vi "Configure.vi"(8 "error in (no error)":errorcluster, 10 "ConfigRef In":T1, 11 "Temperature Device in":refnum<class "Temperature Device.lvclass">) -> (0 "error out":errorcluster, 3 "Temperature Device out":refnum<class "Temperature Device.lvclass">)   [LabVIEW 2015, in "Temperature Device.lvclass"]
uses:
  Temperature Device.lvclass
  <vilib>/Utility/config.llb/Config Data RefNum.ctl
  <vilib>/Utility/config.llb/NI_LVConfig.lvlib
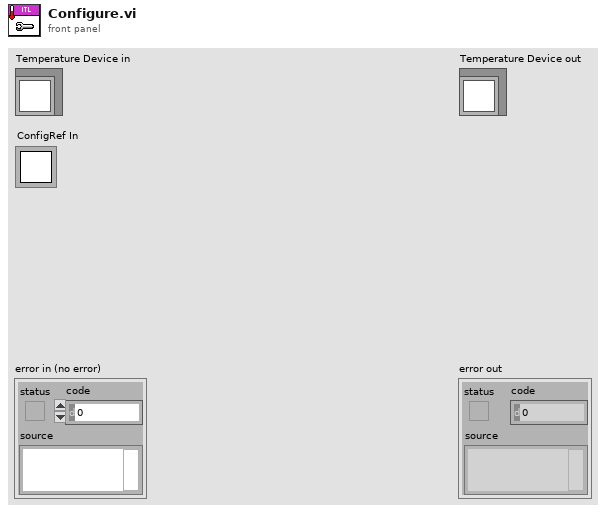
[diagram p1: front panel]
types:
  T1 = typedef "NI_LVConfig.lvlib/Config Data RefNum.ctl" = refnum<k1>
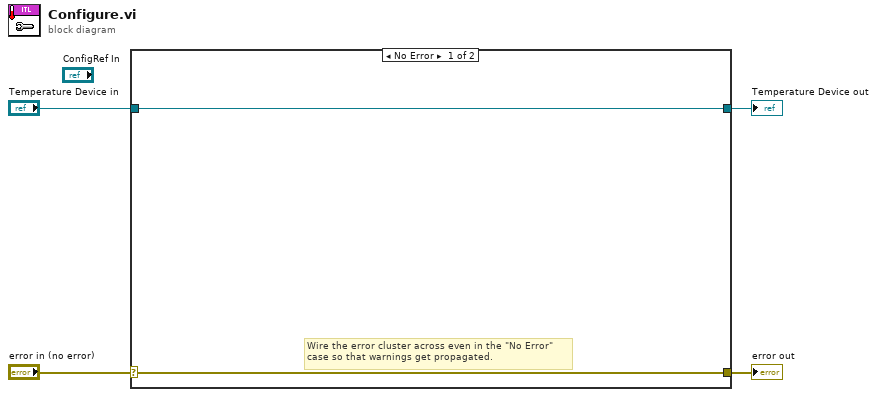
[diagram p0: block diagram]
diagram:
  n1 = case shown="No Error" "error in (no error)" {
    selector: "error in (no error)" -> [w5 w8]
    tunnel: [w5 w8] -> w3
    tunnel: [w6 w7] -> w1
    tunnel: "Temperature Device in" -> [w6 w7]
    frame No Error {
      # "Wire the error cluster across even in the \"No Error\"\ncase so that warnings get propagated."
    }
    frame Error {
    }
  }
  "error out" <- w3
  "Temperature Device out" <- w1
